vi "4-wire xVDT Sim.vi"(0 "Input Channel":refnum<k21>, 1 "Output Channel":refnum<k21>, 2 "xVDT#.Scale1":fxp<+/-,19,5>, 4 "Last Value":i16) -> (5 "Next Value":i16)   [LabVIEW 2010]
uses:
  <vilib>/eio/EIONode/EIONode.xnode
  <vilib>/rvi/eio/nirviEIOImplementation/nirviEIOImplementation.xnode
  <vilib>/rvi/eio/common/nirviEmuClasses.ctl
  <vilib>/rvi/eio/common/nirviEmuTemplateMethod_noerrors.vi
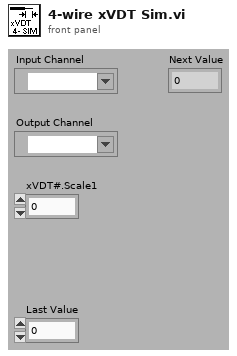
[diagram p1: front panel]
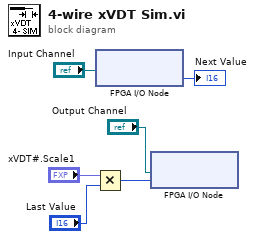
[diagram p0: block diagram]
diagram:
  n1 = Multiply(x="xVDT#.Scale1", y="Last Value") -> (x*y=w1:i16)
  n2 = xnode "FPGA I/O Node"("FPGA I/O In"="Input Channel") -> ("I/O Item"=→"Next Value":i16)  [unwired: 1 out]
  n3 = xnode "FPGA I/O Node"("I/O Item"=w1, "FPGA I/O In"="Output Channel") -> ()  [unwired: 1 out]
